vi "hydrolyse_reactor_repetition_check.vi"(10 "#":i32, 11 "Prior Reactor":refnum<vi>) -> (1 "Prior Path":path, 2 "Current Path":path, 3 "Repetition?":bool)   [LabVIEW 2019]
uses:
  lib/libSimulationControl/libSimulationControl.lvlib
panel:
  # "*******************************************************************\nBiogas Plant Control\n\nAuthor: Paul Zügel\nGCSC-Frankfurt am Main 2020\n\n*******************************************************************"
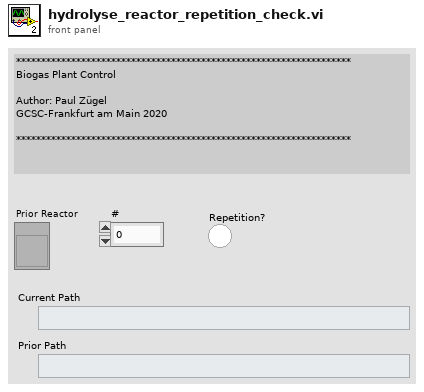
[diagram p1: front panel]
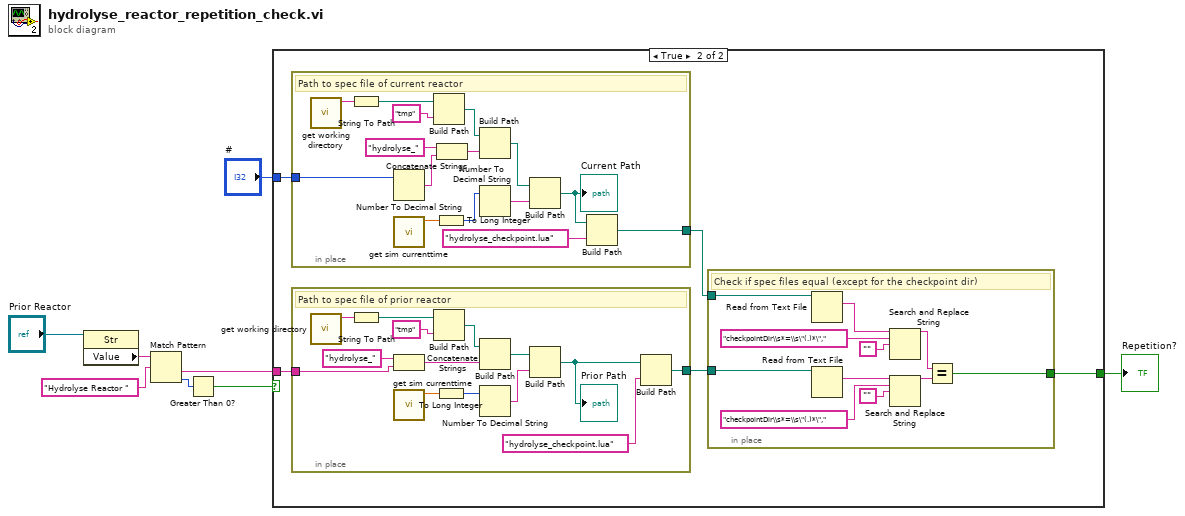
[diagram p0: block diagram]
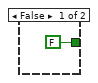
[diagram p2: hidden frame]
diagram:
  n1 = property class="Str"(reference="Prior Reactor") -> ("Value"=w8:string)  [unwired: 1 in, 2 out]
  n2 = Match Pattern(string=w8, regular expression="Hydrolyse Reactor ") -> (after substring=w4:string, offset past match=w6:i32)  [unwired: 1 in, 2 out]
  n3 = Greater Than 0?(x=w6) -> (x > 0?=w5:bool)
  n4 = case shown="True" w5 {
    tunnel: w4 -> [_ w14]
    tunnel: "#" -> [_ w13]
    tunnel: [FALSE w10] -> w1
    frame False {
    }
    frame True {
      n5 = in-place {
        in-place-border: w13 -> [w49]
        in-place-border: [w40] -> w12
        # "Path to spec file of current reactor"
        n6 = call "get working directory.vi"() -> ("function return"=w46:string)  [unwired: 10 in, 1 out]
        n7 = String To Path(string=w46) -> (path=w52:path)
        n8 = Number To Decimal String(number=w49) -> (decimal integer string=w48:string)  [unwired: 1 in]
        n9 = call "get sim currenttime.vi"() -> ("current_time"=w45:dbl)  [unwired: 10 in, 1 out]
        n10 = Build Path(base path=w52, name or relative path="tmp") -> (appended path=w53:path)
        n11 = To Long Integer(number=w45) -> (32bit integer=w44:i32)
        n12 = Concatenate Strings("hydrolyse_" ("string"), w48) -> (w54:string)
        n13 = Build Path(base path=w53, name or relative path=w54) -> (appended path=w47:path)
        n14 = Number To Decimal String(number=w44) -> (decimal integer string=w43:string)  [unwired: 1 in]
        n15 = Build Path(base path=w47, name or relative path=w43) -> (appended path=w42:path)
        "Current Path" <- w42
        n16 = Build Path(base path=w42, name or relative path="hydrolyse_checkpoint.lua") -> (appended path=w40:path)
      }
      n17 = in-place "In Place Element Structure" {
        in-place-border: w14 -> [w34]
        in-place-border: [w26] -> w11
        # "Path to spec file of prior reactor"
        n18 = call "get working directory.vi"() -> ("function return"=w29:string)  [unwired: 10 in, 1 out]
        n19 = String To Path(string=w29) -> (path=w37:path)
        n20 = Concatenate Strings("hydrolyse_" ("string"), w34) -> (w39:string)
        n21 = call "get sim currenttime.vi"() -> ("current_time"=w32:dbl)  [unwired: 10 in, 1 out]
        n22 = Build Path(base path=w37, name or relative path="tmp") -> (appended path=w38:path)
        n23 = To Long Integer(number=w32) -> (32bit integer=w31:i32)
        n24 = Build Path(base path=w38, name or relative path=w39) -> (appended path=w33:path)
        n25 = Number To Decimal String(number=w31) -> (decimal integer string=w30:string)  [unwired: 1 in]
        n26 = Build Path(base path=w33, name or relative path=w30) -> (appended path=w28:path)
        "Prior Path" <- w28
        n27 = Build Path(base path=w28, name or relative path="hydrolyse_checkpoint.lua") -> (appended path=w26:path)
      }
      n28 = in-place {
        in-place-border: w12 -> [w25]
        in-place-border: w11 -> [w24]
        in-place-border: [w23] -> w10
        # "Check if spec files equal (except for the checkpoint dir)"
        n29 = Read from Text File(file (use dialog)=w25) -> (text=w22:string)  [unwired: 3 in, 3 out]
        n30 = Read from Text File(file (use dialog)=w24) -> (text=w19:string)  [unwired: 3 in, 3 out]
        n31 = Search and Replace String(input string=w22, search string="checkpointDir\\s*=\\s\"(.)*\",", replace string="") -> (result string=w15:string)  [unwired: 5 in, 3 out]
        n32 = Search and Replace String(input string=w19, search string="checkpointDir\\s*=\\s\"(.)*\",", replace string="") -> (result string=w16:string)  [unwired: 5 in, 3 out]
        n33 = Equal?(x=w15, y=w16) -> (x = y?=w23:bool)
      }
    }
  }
  "Repetition?" <- w1
